vi "Actor Core.vi"(8 "error in":errorcluster, 11 "Nested Actor in":refnum<class "Nested Actor.lvclass">) -> (0 "error out":errorcluster, 3 "Actor out":refnum<class "Actor.lvclass">)   [LabVIEW 2020, in "Nested Actor.lvlib" / "Nested Actor.lvclass"]
doc: "(<B>Filename</B>: Actor Framework.lvlib:Actor.lvclass:Actor Core.vi)\n\nReceives messages to the actor, reacts to them, and initiates any error handling that may shut the actor down.\n\nDescendant classes may override this VI to append parallel tasks for the actor to complete while it handles messages. Overrides use the Call Parent Class Method node."
uses:
  Nested Actor.lvclass
  C:/Program Files (x86)/National Instruments/LabVIEW 2020/vi.lib/ActorFramework/Actor/Actor.lvclass
  <vilib>/ActorFramework/Actor/Actor.lvclass
  <vilib>/ActorFramework/Actor/Actor.lvclass/Actor.ctl
  <vilib>/ActorFramework/Message Enqueuer/Message Enqueuer.lvclass/Message Enqueuer.ctl
  Nested Actor.lvclass/Nested Actor.ctl
  <vilib>/ActorFramework/Message Enqueuer/Init from Existing Queue.vi
  <vilib>/ActorFramework/Message Enqueuer/Enqueue.vi
  <vilib>/ActorFramework/Stop Msg/Stop Msg.lvclass
  C:/Program Files (x86)/National Instruments/LabVIEW 2020/vi.lib/ActorFramework/Message/Message.lvclass
  <vilib>/ActorFramework/Message Priority Queue/Priority Enqueue.vi
  <vilib>/ActorFramework/Message Enqueuer/Message Enqueuer.lvclass
panel:
  out "Rcv From Root":string
  in  "BT_Send":bool
  in  "Content":string
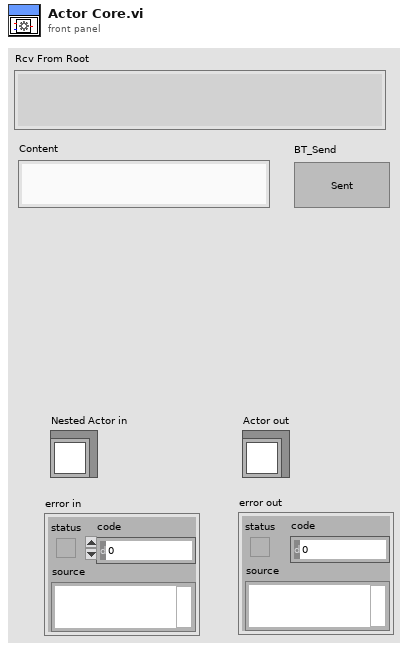
[diagram p1: front panel]
types:
  T1 = cluster{"Stop Event":refnum<user-event>, "Rcv Event":refnum<user-event>}
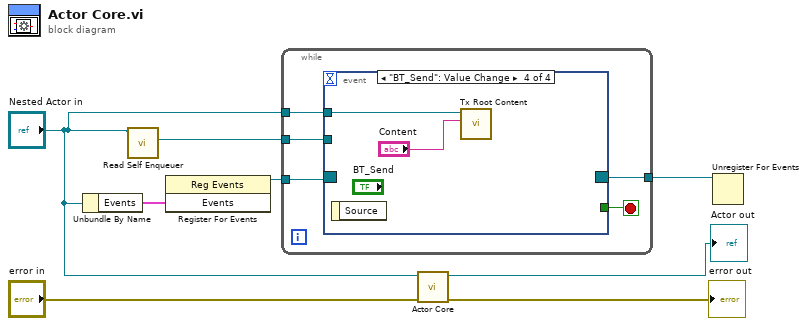
[diagram p0: block diagram]
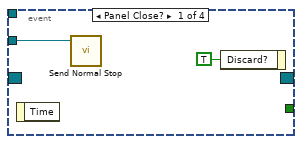
[diagram p2: hidden frame]
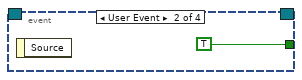
[diagram p3: hidden frame]
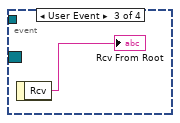
[diagram p4: hidden frame]
diagram:
  n1 = Unbundle By Name("Nested Actor in") -> ("Events"=w5:T1)
  n2 = call <vilib>:"Read Self Enqueuer.vi"("Actor"="Nested Actor in") -> ("Self Enqueuer"=w4:refnum<class "Message Enqueuer.lvclass">)  [unwired: 10 in]
  n3 = register-events(w5) -> (reference out=w3:refnum<event-registration>)  [unwired: 2 in, 1 out]
  n4 = while {
    tunnel: w4 -> [w13]
    tunnel: w3 -> [w12]
    tunnel: [w11] -> w2
    tunnel: "Nested Actor in" -> [w9]
    stop <- w10 stop-if-true
    n5 = event shown="[3] \"BT_Send\": Value Change" {
      selector: w12 -> [_ _ _ _]
      dyn-events: [_ _ _ _] -> w11
      timeout: _ -> [_ _ _ _]
      tunnel: w13 -> [w14 _ _ _]
      tunnel: [_ TRUE _ _] -> w10
      tunnel: w9 -> [_ _ _ w18]
      event Panel Close? {
        n6 = event-data() -> ()  [unwired: 1 in, 1 out]
        n7 = call <vilib>:"Send Normal Stop.vi"("Message Enqueuer"=w14) -> ()  [unwired: 10 in, 1 out]
        n8 = event-data("Discard?"=TRUE) -> ()  [unwired: 1 in, 1 out]
      }
      event User Event {
        n9 = event-data() -> ()  [unwired: 1 in, 1 out]
      }
      event User Event {
        n10 = event-data() -> ("Rcv"=→"Rcv From Root":string)  [unwired: 1 in]
      }
      event "BT_Send": Value Change {
        n11 = event-data() -> ()  [unwired: 1 in, 1 out]
        n12 = call "Tx Root Content.vi"("Content"="Content", "Nested Actor in"=w18) -> ()  [unwired: 8 in, 2 out]
      }
    }
  }
  n13 = call-parent "Actor Core.vi"("error in"="error in", "Actor in"="Nested Actor in") -> ("error out"=→"error out":errorcluster, "Actor out"=→"Actor out":refnum<class "Actor.lvclass">)  [unwired: 8 in]
  n14 = Unregister For Events(event registration refnum=w2) -> ()  [unwired: 1 in, 1 out]
